vi "Memory.Array.Numeric.Write power of 2.vi"(8 "error in (no error)":errorcluster, 10 "power of 2":i16, 11 "Numeric Array in":refnum<class "Memory.Array.Numeric.lvclass">) -> (0 "error out":errorcluster, 3 "Numeric Array out":refnum<class "Memory.Array.Numeric.lvclass">)   [LabVIEW 2016, in "LabVIEW Memory Manager.lvlib" / "Memory.Array.Numeric.lvclass"]
uses:
  Memory.Array.Numeric.lvclass
  Memory.Array.Numeric.lvclass/Memory.Array.Numeric.ctl
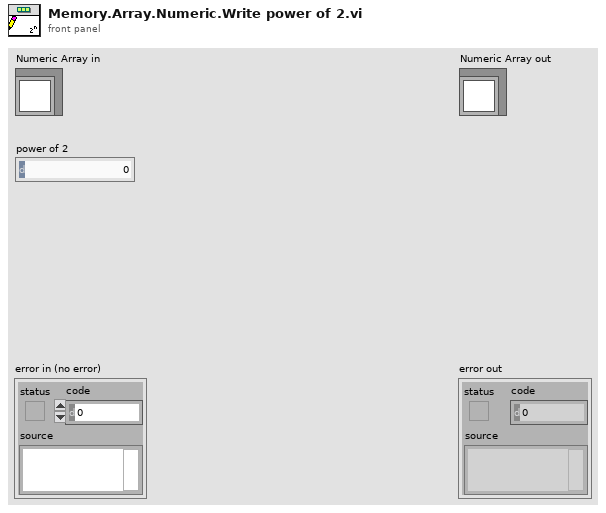
[diagram p1: front panel]
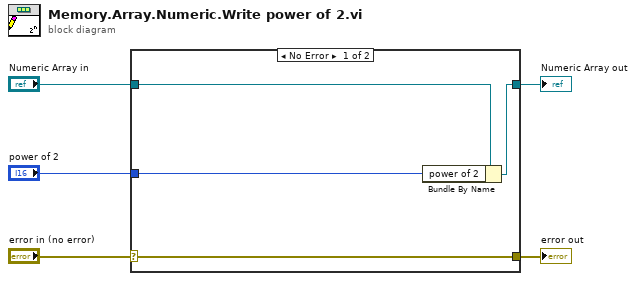
[diagram p0: block diagram]
diagram:
  n1 = case shown="No Error" "error in (no error)" {
    selector: "error in (no error)" -> [w9 w10]
    tunnel: [w9 w10] -> w4
    tunnel: [w7 w11] -> w2
    tunnel: "Numeric Array in" -> [w8 w11]
    tunnel: "power of 2" -> [w6 _]
    frame No Error {
      n2 = Bundle By Name(cluster=w8, "power of 2"=w6) -> (w7:refnum<class "Memory.Array.Numeric.lvclass">)
    }
    frame Error {
    }
  }
  "error out" <- w4
  "Numeric Array out" <- w2
